vi "State Enter Core.vi"(8 "error in (no error)":errorcluster, 11 "A Context State in":refnum<class "A Context State.lvclass">) -> (0 "error out":errorcluster, 3 "A Context State out":refnum<class "A Context State.lvclass">)   [LabVIEW 2021, in "Context.lvlib" / "A Context State.lvclass"]
uses:
  A Context State.lvclass
  A Context State.lvclass/A Context State.ctl
  Context/Context.lvclass
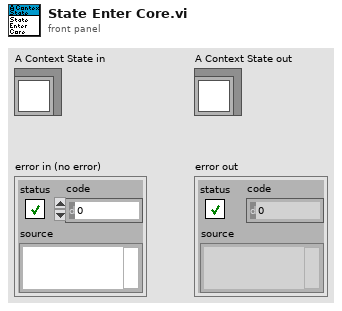
[diagram p1: front panel]
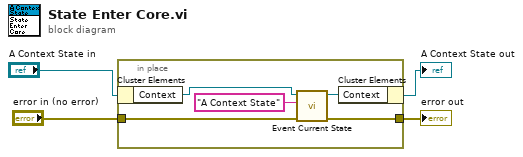
[diagram p0: block diagram]
diagram:
  n1 = in-place {
    in-place-border: "error in (no error)" -> [w7]
    in-place-border: [w6] -> w1
    n2 = in-place-cluster #1("A Context State in") -> ("Context"=w9:refnum<class "Context.lvclass">)
    n3 = call "Event Current State.vi"("error in (no error)"=w7, "Current State"="A Context State", "Context in"=w9) -> ("error out"=w6:errorcluster, "Context out"=w8:refnum<class "Context.lvclass">)  [unwired: 7 in]
    n4 = in-place-cluster #1("Context"=w8) -> (→"A Context State out":refnum<class "A Context State.lvclass">)
  }
  "error out" <- w1
